vi "Send_to_VISA_serial_port.vi"(2 "Error In":errorcluster, 3 "Exiting?":bool, 4 "IO Live params in":T1) -> (0 "Error Out":errorcluster, 1 "IO Live params out":T1)   [LabVIEW 2018, in "TTL IO.lvlib"]
uses:
  TTL IO.lvlib
  Typedefs/CTL_IO_Live_params.ctl
  Typedefs/CTL_IO_action.ctl
  Typedefs/CTL_IO_ports_status.ctl
  Typedefs/CTL_TTL_command_block.ctl
  SubVi's/Controls/CTL_Condition_response_type.ctl
  Common_Resources.lvlib
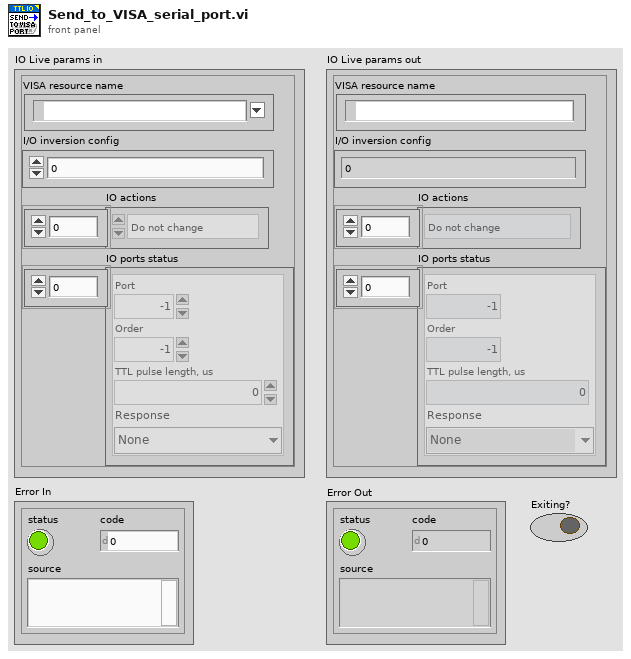
[diagram p1: front panel]
types:
  T1 = typedef "TTL IO.lvlib/CTL_IO_Live_params.ctl" = cluster{"VISA resource name":refnum<visa-resource-name>, "I/O inversion config":u32, "IO actions":T2[], "IO ports status":T3}
  T2 = typedef "TTL IO.lvlib/CTL_IO_action.ctl" = enum16{"Do not change", "Fire up", "Shut down"}
  T3 = typedef "TTL IO.lvlib/CTL_IO_ports_status.ctl" = T4[]
  T4 = typedef "TTL IO.lvlib/CTL_TTL_command_block.ctl" = cluster{"Port":i16, "Order":i32, "TTL pulse length, us":i32, "Response":T5}
  T5 = typedef "Common_Resources.lvlib/CTL_Condition_response_type.ctl" = enum16{"None", "Air puff", "Liquid reward", "TTL pulse", "TTL pulse (ubr)", "TTL signal"}
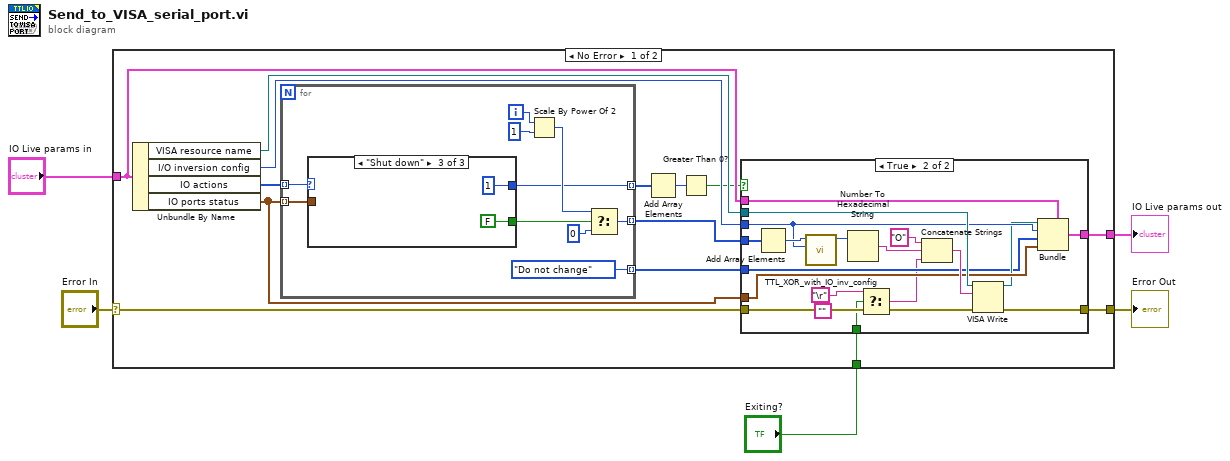
[diagram p0: block diagram]
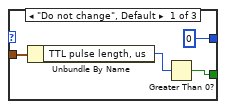
[diagram p3: hidden frame]
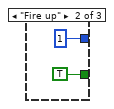
[diagram p4: hidden frame]
diagram:
  n1 = case shown="No Error" "Error In" {
    selector: "Error In" -> [w19 w60]
    tunnel: [w18 w60] -> w4
    tunnel: "IO Live params in" -> [w12 w59]
    tunnel: [w10 w59] -> w2
    tunnel: "Exiting?" -> [w6 _]
    frame No Error {
      n2 = Unbundle By Name(w12) -> ("VISA resource name"=w16:refnum<visa-resource-name>, "I/O inversion config"=w15:u32, "IO actions"=w14:T2[], "IO ports status"=w13:T3)
      n3 = for {
        tunnel: w14 -> [w50] mode=indexing
        tunnel: w13 -> [w49] mode=indexing
        tunnel: [CTL_IO_action."Do not change" ("IO action")] -> w11 mode=indexing
        tunnel: [w43] -> w17 mode=indexing
        tunnel: [w41] -> w9 mode=indexing
        i -> [w47]
        n4 = case shown="\"Shut down\"" w50 {
          tunnel: w49 -> [w54 _ _]
          tunnel: [w52 TRUE FALSE] -> w45
          tunnel: [0 1 1] -> w41
          frame "Do not change", Default {
            n5 = Unbundle By Name(w54) -> ("TTL pulse length, us"=w53:i32)
            n6 = Greater Than 0?(x=w53) -> (x > 0?=w52:bool)
          }
          frame "Fire up" {
          }
          frame "Shut down" {
          }
        }
        n7 = Scale By Power Of 2(n=w47, x=u8 1) -> (x*2^n=w44:u8)
        n8 = Select(t=w44, s=w45, f=u8 0) -> (s? t:f=w43:u8)
      }
      n9 = Add Array Elements(numeric array=w9) -> (sum=w8:i32)
      n10 = Greater Than 0?(x=w8) -> (x > 0?=w7:bool)
      n11 = case shown="True" w7 {
        tunnel: w19 -> [w20 w37]
        tunnel: [w20 w35] -> w18
        tunnel: w17 -> [_ w34]
        tunnel: w16 -> [_ w32]
        tunnel: w15 -> [_ w31]
        tunnel: w13 -> [_ w30]
        tunnel: w12 -> [w21 w29]
        tunnel: w11 -> [_ w27]
        tunnel: [w21 w26] -> w10
        tunnel: w6 -> [_ w22]
        frame False {
        }
        frame True {
          n12 = Add Array Elements(numeric array=w34) -> (sum=w33:u8)
          n13 = call "TTL_XOR_with_IO_inv_config.vi"("IO inversion config."=w31, "Ports config to fire"=w33) -> ("ON config."=w38:u32)  [unwired: 9 in]
          n14 = Number To Hexadecimal String(2:w38) -> (0:w40:string)  [unwired: 1 in]
          n15 = Select(t="\r", s=w22, f="") -> (s? t:f=w25:string)
          n16 = Concatenate Strings("O" ("string"), w40, w25) -> (w36:string)
          n17 = VISA Write(VISA resource name=w32, write buffer=w36, error in (no error)=w37) -> (VISA resource name out=w28:refnum<visa-resource-name>, error out=w35:errorcluster)  [unwired: 1 out]
          n18 = Bundle(cluster=w29, "VISA resource name"=w28, "I/O inversion config"=w31, "IO actions"=w27, "IO ports status"=w30) -> (w26:T1)
        }
      }
    }
    frame Error {
    }
  }
  "Error Out" <- w4
  "IO Live params out" <- w2
